vi "Set Or Get ActiveCell Font.vi"(6 "Active Cell":T1 caption="活动单元格:活动单元格", 8 "error in (no error)":errorcluster caption="错误输入（无错误）", 9 "Mode":T3, 10 "CellFont In":T2 caption="CellFont", 11 "Table Ref In":refnum<vi>) -> (0 "error out":errorcluster caption="错误输出", 2 "CellFont Out":T2 caption="CellFont", 3 "Table Ref Out":refnum<vi>)   [LabVIEW 2013, in "Table Tool.lvlib"]
uses:
  Table Tool.lvlib
  Custum Type/GetOrSet.ctl
  <vilib>/Utility/miscctls.llb/LVFontTypeDef.ctl
  <vilib>/Utility/miscctls.llb/LVRowAndColumnTypeDef.ctl
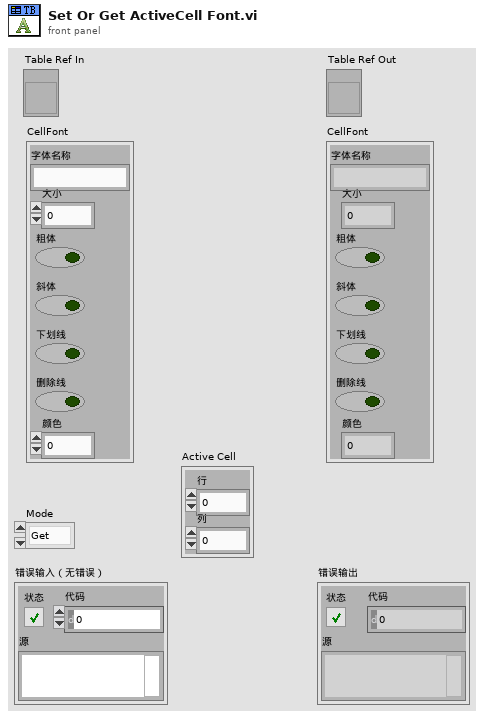
[diagram p1: front panel]
types:
  T1 = typedef "LVRowAndColumnTypeDef.ctl" = cluster{"Row":i32, "Column":i32}
  T2 = typedef "LVFontTypeDef.ctl" = cluster{"Font Name":string, "Size":u16, "Bold":bool, "Italic":bool, "Underline":bool, "Strikeout":bool, "Color":u32}
  T3 = typedef "Table Tool.lvlib/GetOrSet.ctl" = enum16{"Get", "Set"}
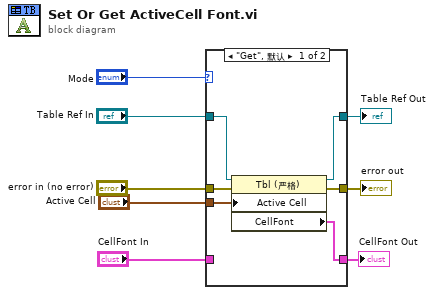
[diagram p0: block diagram]
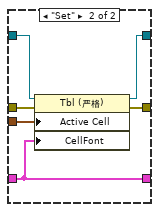
[diagram p2: hidden frame]
diagram:
  n1 = case shown="\"Get\", 默认" "Mode" {
    tunnel: "Table Ref In" -> [w14 w19]
    tunnel: "error in (no error)" -> [w13 w20]
    tunnel: [w12 w17] -> w5
    tunnel: [w11 w18] -> w4
    tunnel: [w9 w15] -> w3
    tunnel: "CellFont In" -> [_ w15]
    tunnel: "Active Cell" -> [w10 w16]
    frame "Get", Default {
      n2 = property class="Tbl (严格)"(reference=w14, error in=w13, "Active Cell"=w10) -> (reference out=w11:refnum<vi>, error out=w12:errorcluster, "CellFont"=w9:T2)
    }
    frame "Set" {
      n3 = property class="Tbl (严格)"(reference=w19, error in=w20, "Active Cell"=w16, "CellFont"=w15) -> (reference out=w18:refnum<vi>, error out=w17:errorcluster)
    }
  }
  "Table Ref Out" <- w4
  "error out" <- w5
  "CellFont Out" <- w3
